vi "Create New Project.vi"(7 "Status Indicator Ref":refnum<vi>, 8 "error in (no error)":errorcluster, 10 "File Path to Append":path, 11 "Build Specs Folder Path":path=path "C:/sw-deps-monitor/Source/BuildSpecs") -> (0 "error out":errorcluster, 3 "Project Created":path)   [LabVIEW 2019, in "Hawkeye.lvlib"]
uses:
  Hawkeye.lvlib
  <userlib>/_OpenG.lib/file/file.llb/Compare Two Paths - Scalar__ogtk.vi
  <userlib>/_OpenG.lib/file/file.llb/File Exists - Scalar__ogtk.vi
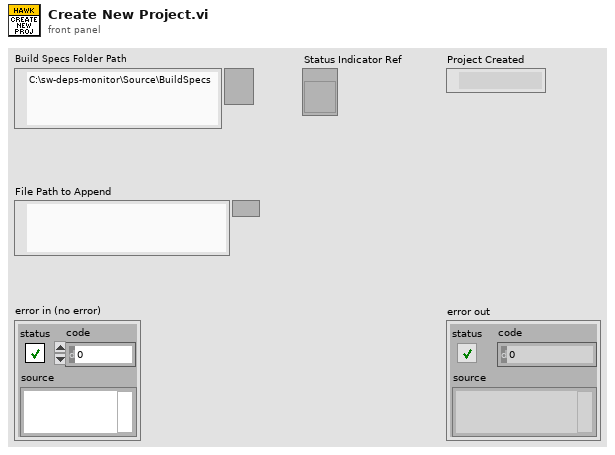
[diagram p1: front panel]
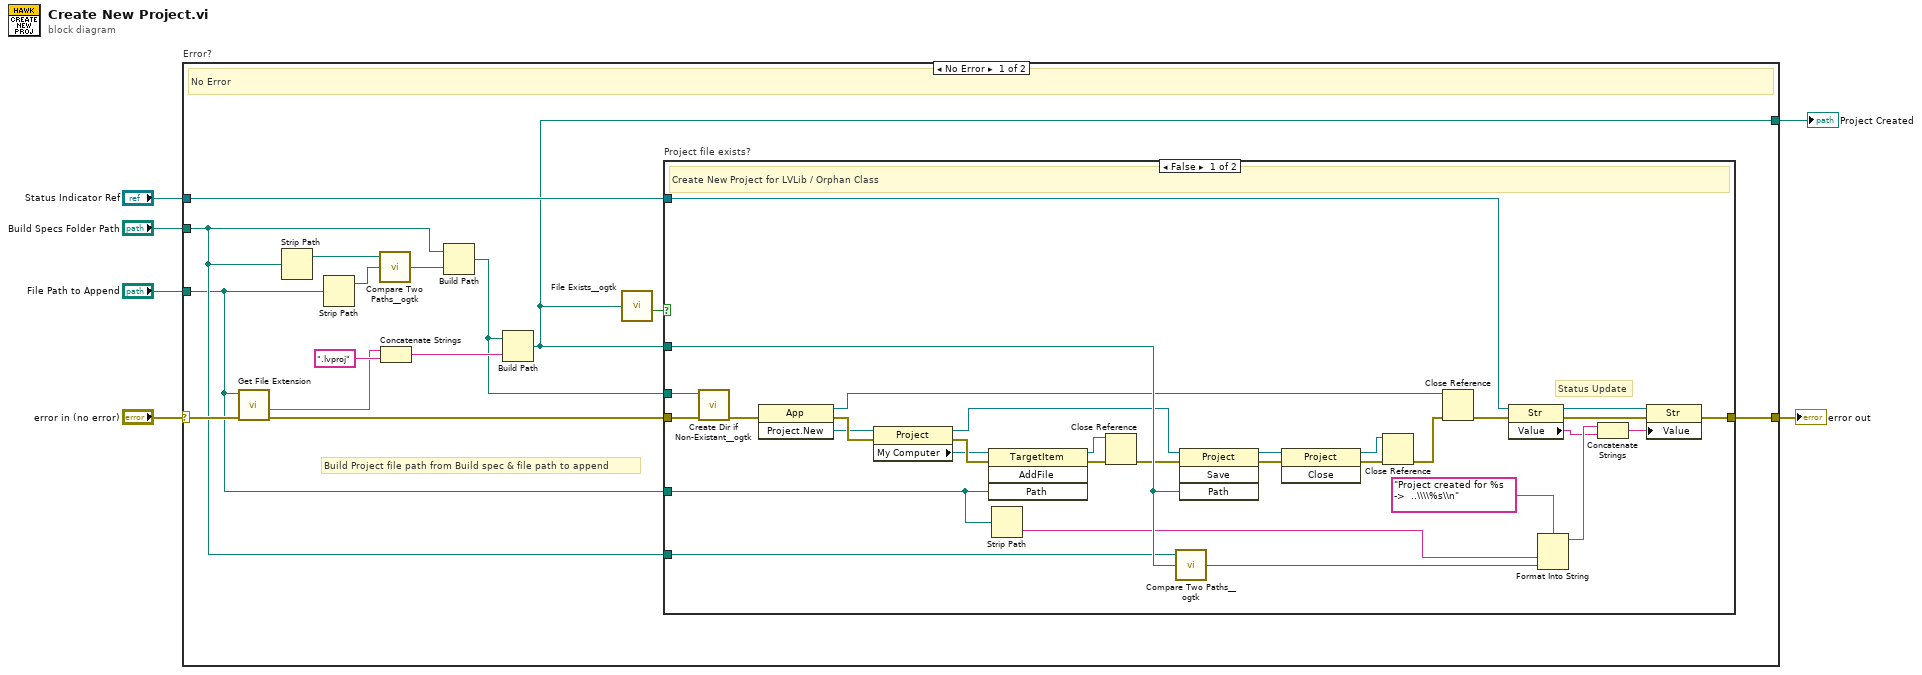
[diagram p0: block diagram]
diagram:
  n1 = case "Error?" shown="No Error" "error in (no error)" {
    selector: "error in (no error)" -> [w21 w54]
    tunnel: "Build Specs Folder Path" -> [w13 _]
    tunnel: [w12 w54] -> w4
    tunnel: "Status Indicator Ref" -> [w11 _]
    tunnel: "File Path to Append" -> [w10 _]
    tunnel: [w8 _] -> w1
    frame No Error {
      # "Build Project file path from Build spec & file path to append"
      # "No Error"
      n2 = call <vilib>:"Get File Extension.vi"("error in (no error)"=w21, "file"=w10) -> ("error out"=w15:errorcluster, "filename without extension"=w18:string)  [unwired: 5 in, 3 out]
      n3 = Strip Path(path=w13) -> (stripped path=w17:path)  [unwired: 1 out]
      n4 = Strip Path(path=w10) -> (stripped path=w9:path)  [unwired: 1 out]
      n5 = call-poly <userlib>:"Compare Two Paths__ogtk.vi"("path2"=w9, "path1"=w17) -> ("relative path from 1 to 2"=w16:path)  [unwired: 1 in, 2 out]
      n6 = Concatenate Strings(w18, ".lvproj" ("string")) -> (w19:string)
      n7 = Build Path(base path=w13, name or relative path=w16) -> (appended path=w14:path)
      n8 = Build Path(base path=w14, name or relative path=w19) -> (appended path=w8:path)
      n9 = call-poly <userlib>:"File Exists__ogtk.vi"("file path"=w8) -> ("exists"=w7:bool)  [unwired: 6 in, 1 out]
      n10 = case "Project file exists?" shown="False" w7 {
        tunnel: w8 -> [w52 _]
        tunnel: w15 -> [w31 w53]
        tunnel: w14 -> [w30 _]
        tunnel: w13 -> [w29 _]
        tunnel: [w28 w53] -> w12
        tunnel: w11 -> [w27 _]
        tunnel: w10 -> [w26 _]
        frame False {
          # "Status Update"
          # "Create New Project for LVLib / Orphan Class"
          n11 = call <userlib>:"Create Dir if Non-Existant__ogtk.vi"("error in (no error)"=w31, "Directory Path"=w30) -> ("error out"=w32:errorcluster)  [unwired: 7 in, 2 out]
          n12 = invoke on="Invoke Node" class="App" method="Project.New"(error in=w32) -> (reference out=w42:refnum<vi>, error out=w43:errorcluster, "Project:New"=w41:refnum<vi>)  [unwired: 2 in]
          n13 = property on="Property Node" class="Project"(reference=w41, error in=w43) -> (reference out=w49:refnum<vi>, error out=w45:errorcluster, "My Computer"=w44:refnum<vi>)
          n14 = invoke on="Invoke Node" class="TargetItem" method="AddFile"(reference=w44, error in=w45, "Path"=w26) -> (reference out=w46:refnum<vi>, error out=w47:errorcluster)  [unwired: 1 in, 2 out]
          n15 = Strip Path(path=w26) -> (name=w36:string)  [unwired: 1 out]
          n16 = Close Reference(reference=w46, error in (no error)=w47) -> (error out=w33:errorcluster)
          n17 = call-poly <userlib>:"Compare Two Paths__ogtk.vi"("path2"=w52, "path1"=w29) -> ("relative path from 1 to 2"=w34:path)  [unwired: 1 in, 2 out]
          n18 = invoke on="Invoke Node" class="Project" method="Save"(reference=w49, error in=w33, "Path"=w52) -> (reference out=w23:refnum<vi>, error out=w50:errorcluster)  [unwired: 1 in, 2 out]
          n19 = invoke class="Project" method="Close"(reference=w23, error in=w50) -> (reference out=w22:refnum<vi>, error out=w24:errorcluster)  [unwired: 1 in, 1 out]
          n20 = Close Reference(reference=w22, error in (no error)=w24) -> (error out=w48:errorcluster)
          n21 = Close Reference(reference=w42, error in (no error)=w48) -> (error out=w51:errorcluster)
          n22 = property on="Property Node" class="Str"(reference=w27, error in=w51) -> (reference out=w39:refnum<vi>, error out=w40:errorcluster, "Value"=w25:string)
          n23 = Format Into String(format string="Project created for %s  ->  ..\\\\%s\\n", w36, w34) -> (resulting string=w35:string)  [unwired: 2 in, 1 out]
          n24 = Concatenate Strings(w35, w25) -> (w38:string)
          n25 = property on="Property Node" class="Str"(reference=w39, error in=w40, "Value"=w38) -> (error out=w28:errorcluster)  [unwired: 1 out]
        }
        frame True {
          # "Project file found - skipped new project creation"
        }
      }
    }
    frame Error {
      # "Error Found Skip the process"
    }
  }
  "error out" <- w4
  "Project Created" <- w1
